vi "FFT -- V2.vi"() -> ()   [LabVIEW 2021]
uses:
  fft -- data win.ctl
  cursor winow sygnal plot.ctl
  cursor window action.ctl
  <vilib>/measure/maspectr.llb/FFT Power Spectrum for N Chan.vi
  <vilib>/measure/NI_MAPro.lvlib
panel:
  in  "landscape":enum32{"Page 1", "Page 2"}(tab)
  in  "scan step":dbl=0.0001 format="%#_3p"
  in  "accumulate":bool
  in  "clear":bool
  in  "update":bool
  out "landscape plot":cluster{dbl[], dbl[]}[](graph)
  in  "offset":dbl(slide)=5968.8832085721915 scale=50.0..50000.0 scale format="%#_3p"
  out "N":dbl=1.0
  in  "scan":bool
  in  "Tab Control":enum32{"Page 1", "Page 2"}(tab)
  in  "Input file path":path=path "/Users/arkadyshekhter/Desktop/gdrive/data/Vikram&Shiva&Zoltan--Aug2025/August_2025/082225/p_c4_006_082225.tdms"
  out "FFT Graph":cluster{"f0":dbl, "df":dbl, "magnitude":dbl[]}[](graph)=[{"f0"=0.0, "df"=323.0255868567349, "magnitude"=array[4691 elements]}]
  out "Signal graph":waveform(dbl)[](graph)=[{"t0"=timestamp(-0.009969989999999984 s since 1904-01-01), "dt"=3.3e-07, "Y"=array[333333 elements], "attributes"=variant("Configuration"=variant(string "[Configuration]\nConfiguration.Post-trigger delay = \"-0.010000000000\"\nConfiguration.Post-trigger duration = \"0.10000000000\"\nConfiguration.Rate = \"3030303.0303\"\nConfiguration.Ranges = \"<size(s)=5> 10.000000000 10.000000000 10.000000000 1.0000000000 1.0000000000\"\nConfiguration.Re-name channels.<size(s)> = \"5\"\nConfiguration.Re-name channels 0 = \"Idot\"\nConfiguration.Re-name channels 1 = \"Bdot\"\nConfiguration.Re-name channels 2 = \"Bproj\"\nConfiguration.Re-name channels 3 = \"freq\"\nConfiguration.Re-name channels 4 = \"drive\"\nConfiguration.Active channels = \"0,1,2,5,6\"\nConfiguration.External\\nclock = \"FALSE\"\nConfiguration.Monitor time\\nconstant = \"1.0000000000\"\nConfiguration.Sync = \"TRUE\"\nConfiguration.Lock-in input channel phases = \"<size(s)=0> \"\nConfiguration.Output channels configuration.<size(s)> = \"0\""), "NI_ChannelName"=variant(string "freq"))}]
  in  "Data window":T1={"Start"=58340, "Length"=9381, "Channel numbers"=[0], "Cannel names"=["freq", ""], "Group name"="p"}
  in  "run":bool
  out "dt (sec)":dbl=3.3e-07
  in  "digitiz. freq (Hz)":dbl=3000000.0 format="%#_3p"
  out "win (sec)":dbl=0.003127 format="%#_3p"
  out "time (sec)":dbl=0.020800065 format="%#_3p"
  in  "signal cursor":T2={"left"=0.01944671559633024, "right "=0.02257377719528174, "center"=0.02101024639580599, "window"=0.0031270615989515034, "cursors"=[0, 1, 2], "relative"=0, "absolute"=0, "fixed vertical offset"=0.0, "vertical offset"=0.0, "skew"=0.0, "default window frac"=0.1, "kind"=enum."symmetric", "skew.left"=0.5, "skew.right"=0.5, "wing order"=enum."back", "Plot ref Syg"=refnum}
  out "scan times":dbl[](array[numeric])
  out "XY Graph":cluster{dbl[], dbl[]}(graph)
  # "OR"
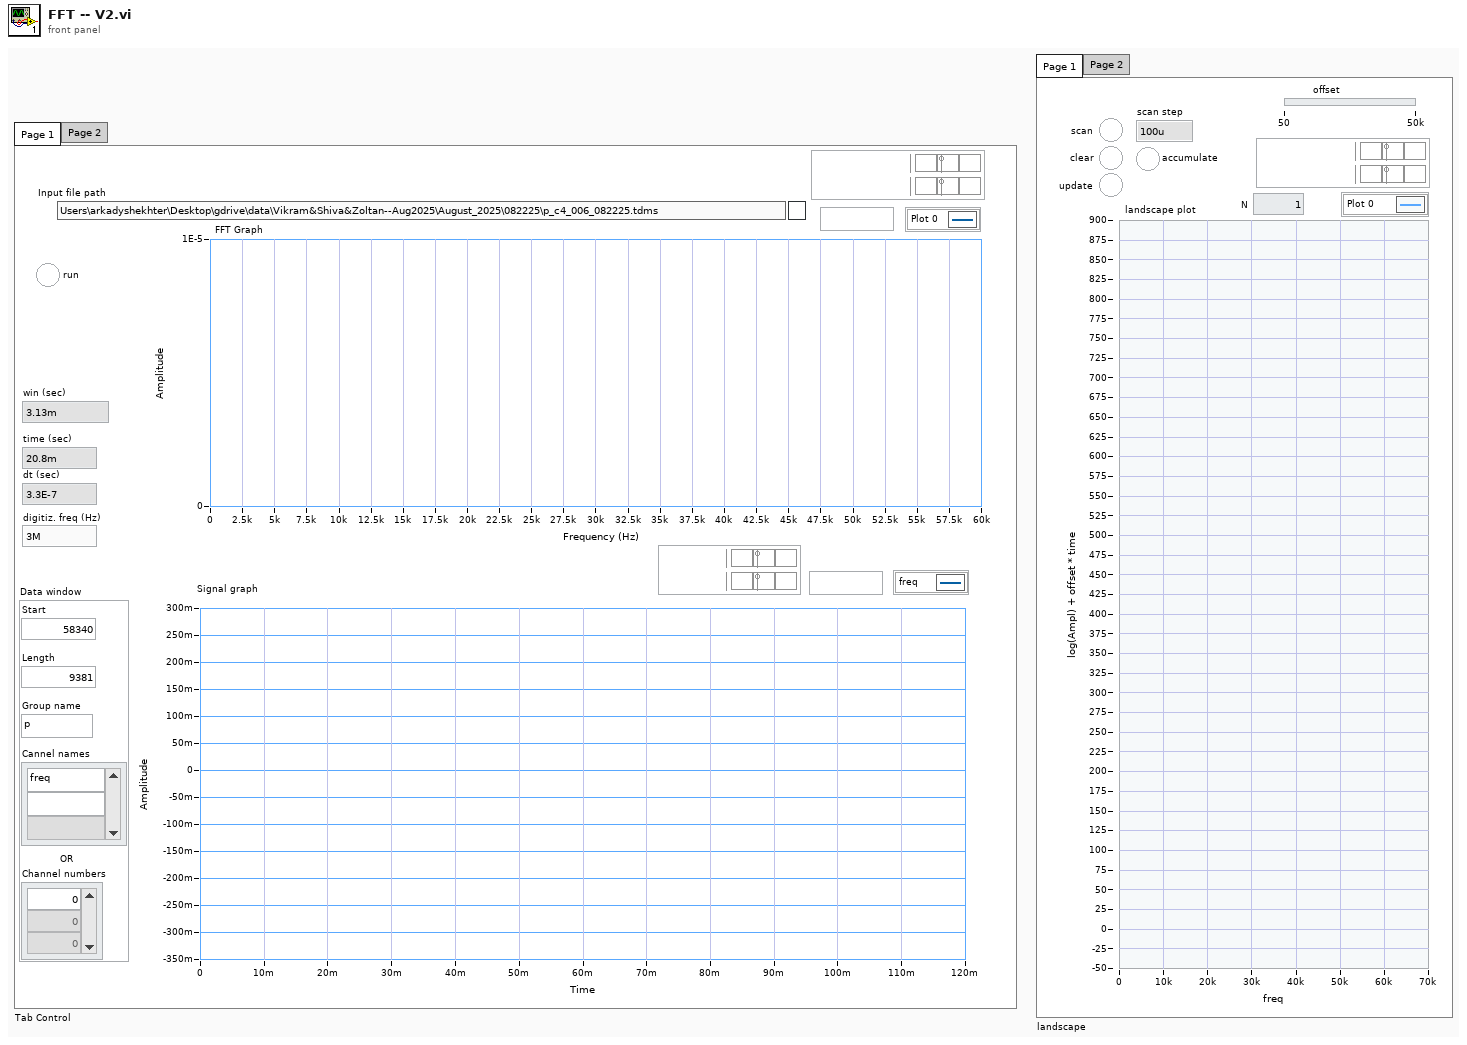
[diagram p1: front panel]
types:
  T1 = typedef "fft -- data win.ctl" = cluster{"Start":i64, "Length":i32, "Channel numbers":i64[], "Cannel names":string[], "Group name":string}
  T2 = typedef "cursor winow sygnal plot.ctl" = cluster{"left":dbl, "right ":dbl, "center":dbl, "window":dbl, "cursors":i32[], "relative":i32, "absolute":i32, "fixed vertical offset":dbl, "vertical offset":dbl, "skew":dbl, "default window frac":dbl, "kind":enum16{"symmetric", "skewed", "fancy"}, "skew.left":dbl, "skew.right":dbl, "wing order":enum16{"forw", "back"}, "Plot ref Syg":refnum<vi>}
  T3 = typedef "cursor window action.ctl" = enum16{"balance", "h. offset change", "cursor moves", "change center", "change window", "init", "check", "reset", "set y to middle", "idle", "-write all Y", "-write left.X", "-write center.X", "-write right.X", "-write all X", "-change center", "-change window", "-change skew", "-read cursor 2", "-read cursor 1", "-read cursor 0", "-read all cursors", "-reset", "-read plot scale", "-set y to middle", "-Q: center.Y is visible", "-Q: window is visible", "-parse center.Y", "-right left from center", "-left move", "-right move", "-set center.Y", "-empty", "-set cursors to default", "-check", "-write center.Y", "-copy cursor 1", "-copy cursor 0", "-copy cursor 2", "move right", "move left", "shrink", "broaden", "skew up", "skew down", "-write plot scale", "zoom X", "change cen&win", "zoom to all data", "color--red", "color--green", "color--yellow", "read", "zoom out", "zoom in", "slide right", "slide left", "set range aspect ratio to 1", "move to window range", "--move to window range"}
  T4 = enum16{"TDMS file", "Tektronics ISF", "BinF file", "ASCII File", "BinH File", "BinW File", "BINARY File"}
  T5 = typedef "eventvkey.ctl" = enum16{"ASCII", "Enter", "Return", "Shift", "Ctrl", "Alt", "Cmd", "Opt", "Caps", "NumLock", "Clear", "Break", "Up", "Down", "Left", "Right", "Insert", "Delete", "Home", "End", "PageUp", "PageDown", "Escape", "Help", "Pause", "ScrollLock", "F1", "F2", "F3", "F4", "F5", "F6", "F7", "F8", "F9", "F10", "F11", "F12", "F13", "F14", "F15", "F16", "F17", "F18", "F19", "F20", "F21", "F22", "F23", "F24", "Play", "VolumeUp", "VolumeDown", "Mute", "Two Byte Char"}
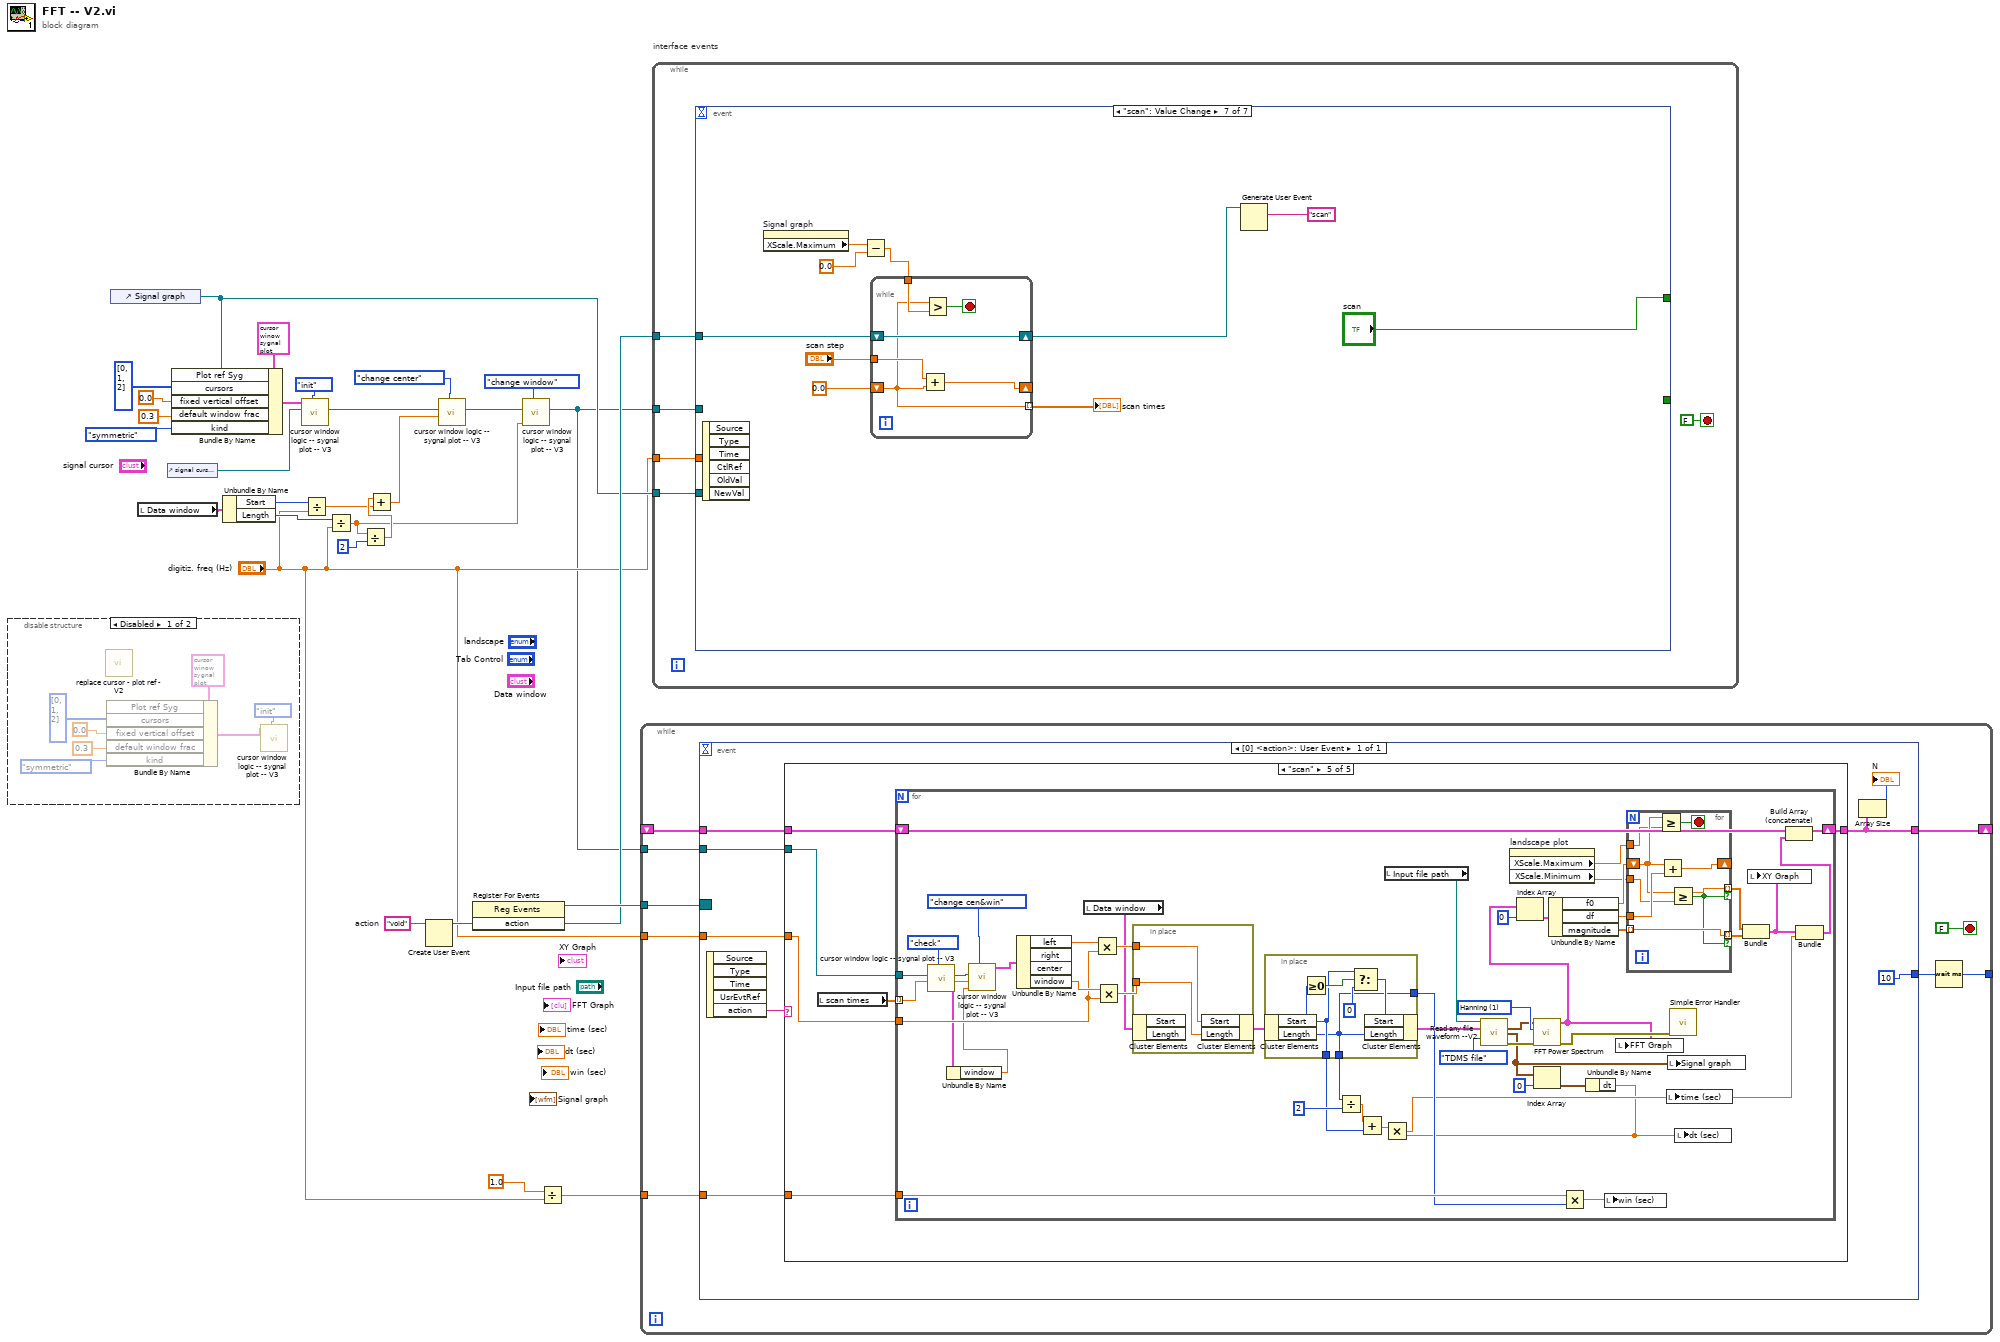
[diagram p0: block diagram]
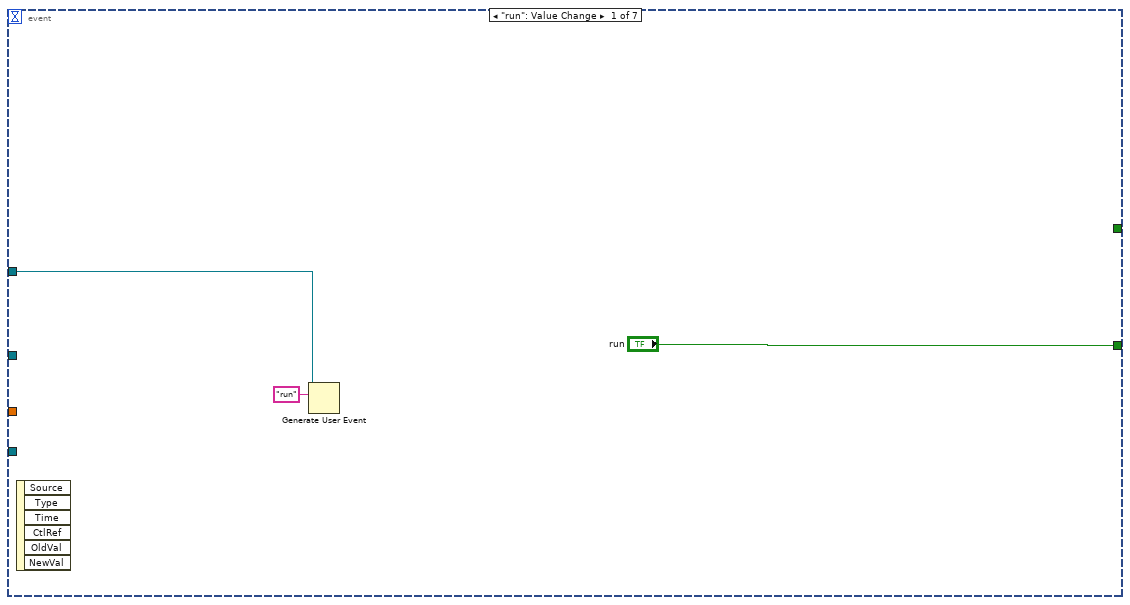
[diagram p3: hidden frame]
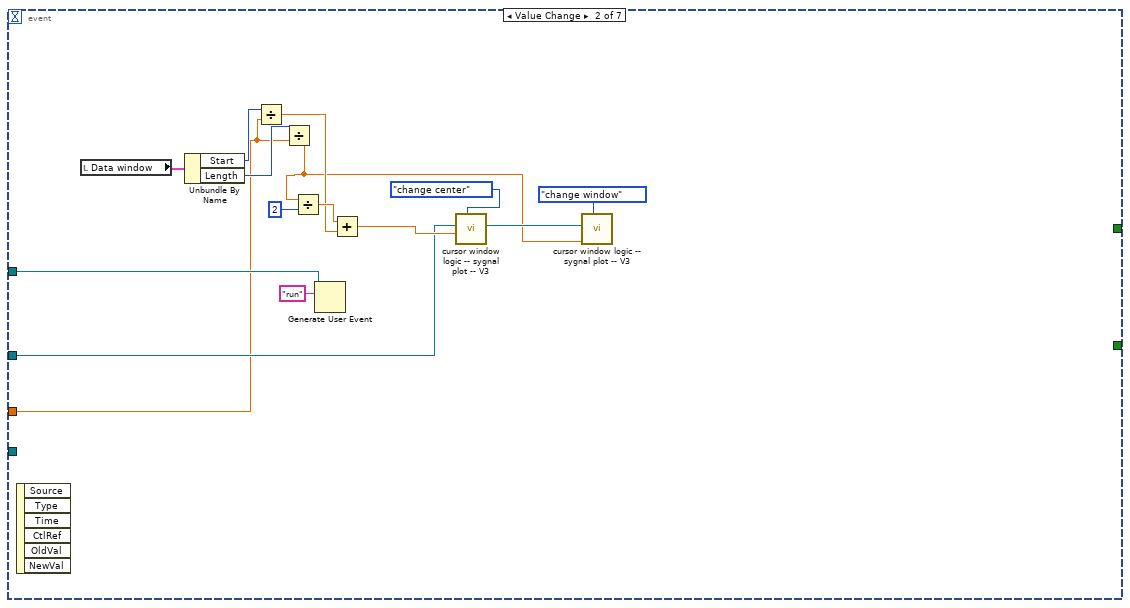
[diagram p4: hidden frame]
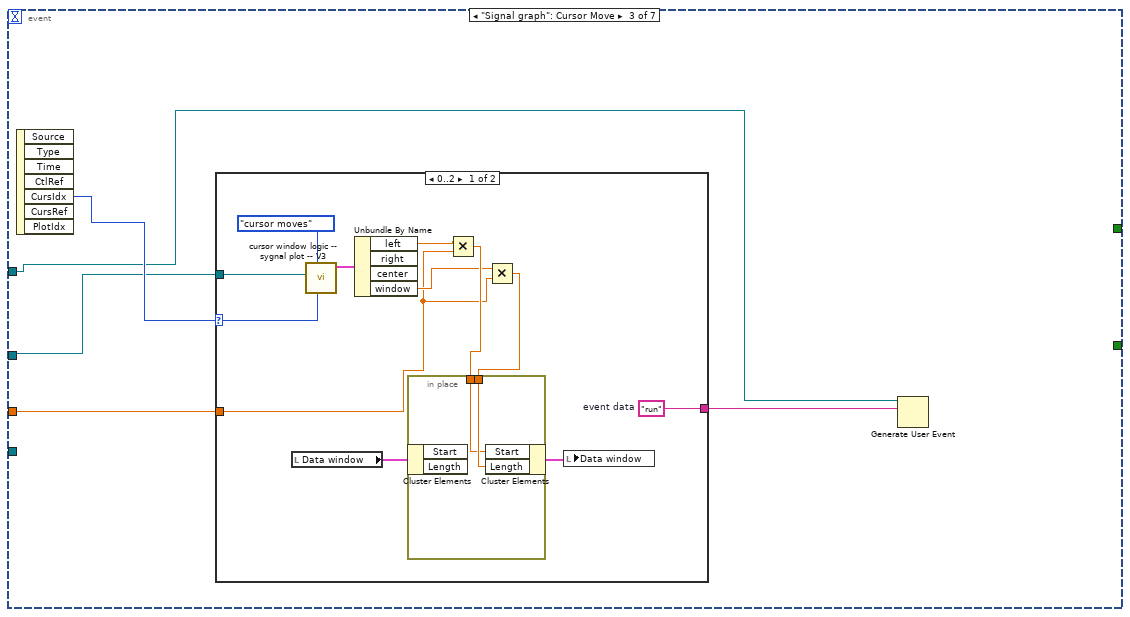
[diagram p5: hidden frame]
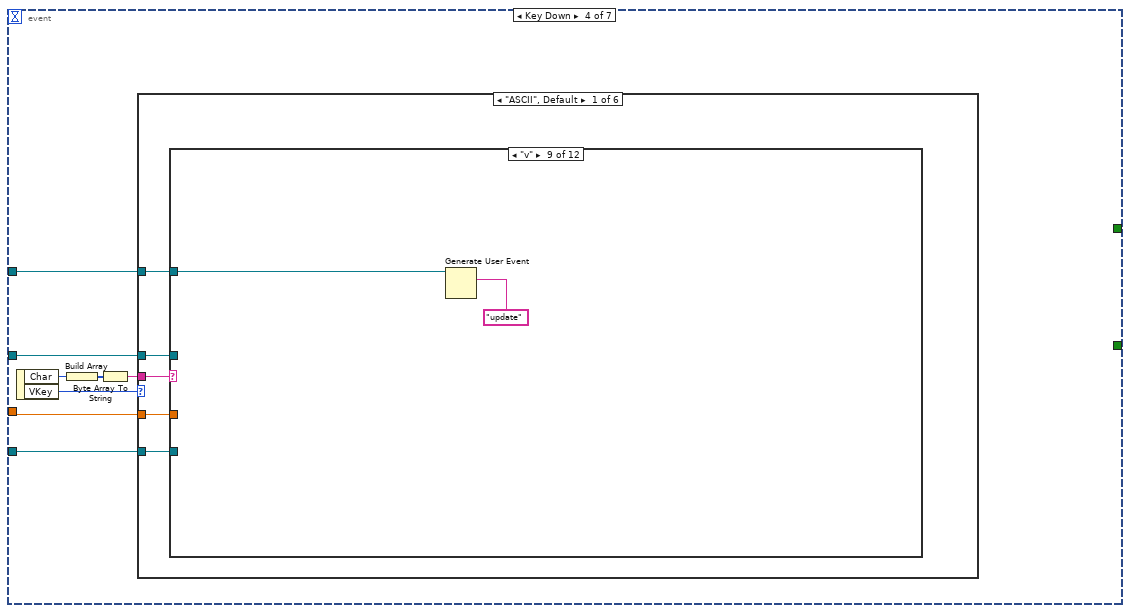
[diagram p7: hidden frame]
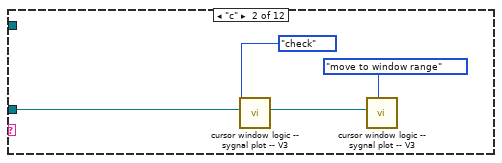
[diagram p9: hidden frame]
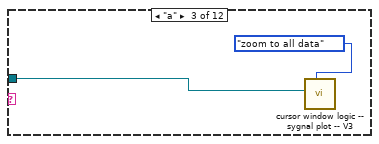
[diagram p10: hidden frame]
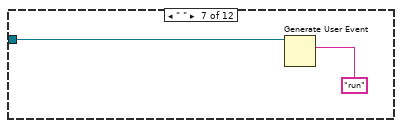
[diagram p14: hidden frame]
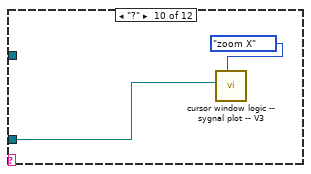
[diagram p16: hidden frame]
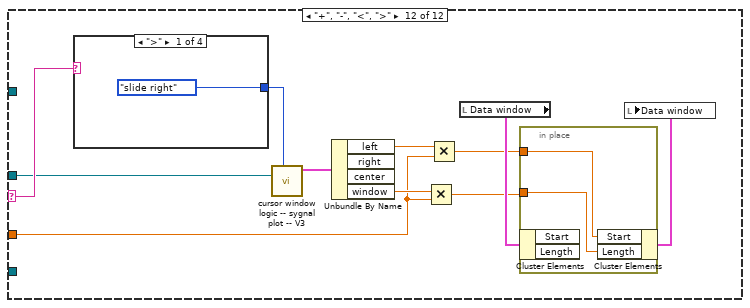
[diagram p18: hidden frame]
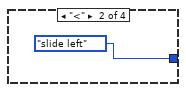
[diagram p19: hidden frame]
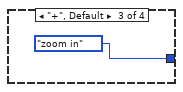
[diagram p20: hidden frame]
diagram:
  w28 = "void"  # action
  n1 = disable-structure shown="Disabled" {
    frame Disabled {
      n2 = call "replace cursor - plot ref - V2.vi"() -> ()  [unwired: 16 in, 4 out]
      n3 = Bundle By Name(cluster=T2 {"left"=2378.60310421286, "right "=2421.6740576496672, "center"=2421.6740576496672, "window"=2421.6740576496672, "cursors"=[], "relative"=0, "absolute"=0, "fixed vertical offset"=2421.6740576496672, "vertical offset"=2421.6740576496672, "skew"=2421.6740576496672, "default window frac"=2421.6740576496672, "kind"=enum."skewed", "skew.left"=2421.6740576496672, "skew.right"=2421.6740576496672, "wing order"=enum."back", "Plot ref Syg"=refnum} ("cursor bracket: All, data window"), "cursors"=i32[] [0, 1, 2], "fixed vertical offset"=0.0, "default window frac"=0.3 ("fixed vertical offset"), "kind"=enum16{"symmetric", "skewed", "fancy"}."symmetric") -> (w29:T2)  [unwired: 1 in]
      n4 = call "cursor window logic -- sygnal plot -- V3.vi"("cursor window action"=cursor_window_action."init", "cursor window init"=w29) -> ()  [unwired: 8 in, 2 out]
    }
    frame Enabled {
    }
  }
  n5 = control-ref of="Signal graph"() -> (w17:refnum<vi>)
  n6 = local read "Data window"() -> (w4:T1)
  n7 = control-ref of="signal cursor ref"() -> (w18:refnum<vi>)
  n8 = Bundle By Name(cluster=T2 {"left"=2378.60310421286, "right "=2421.6740576496672, "center"=2421.6740576496672, "window"=2421.6740576496672, "cursors"=[], "relative"=0, "absolute"=0, "fixed vertical offset"=2421.6740576496672, "vertical offset"=2421.6740576496672, "skew"=2421.6740576496672, "default window frac"=2421.6740576496672, "kind"=enum."skewed", "skew.left"=2421.6740576496672, "skew.right"=2421.6740576496672, "wing order"=enum."back", "Plot ref Syg"=refnum} ("cursor bracket: All, data window"), "Plot ref Syg"=w17, "cursors"=i32[] [0, 1, 2], "fixed vertical offset"=0.0, "default window frac"=0.3 ("fixed vertical offset"), "kind"=enum16{"symmetric", "skewed", "fancy"}."symmetric") -> (w21:T2)
  n9 = Unbundle By Name(w4) -> ("Start"=w5:i64, "Length"=w8:i32)
  n10 = call "cursor window logic -- sygnal plot -- V3.vi"("cursor window action"=cursor_window_action."init", "cursor window IN"=w18, "cursor window init"=w21) -> ("cursor window OUT"=w3:refnum<vi>)  [unwired: 7 in, 1 out]
  n11 = Divide(x=w5, y="digitiz. freq (Hz)") -> (x/y=w7:dbl)
  n12 = Divide(x=w8, y="digitiz. freq (Hz)") -> (x/y=w6:dbl)
  n13 = Divide(x=w6, y=2) -> (x/y=w10:dbl)
  n14 = Add(x=w10, y=w7) -> (x+y=w9:dbl)
  n15 = Create User Event(user event datatype=w28) -> (user event=w26:refnum<user-event>)  [unwired: 1 in, 1 out]
  n16 = call "cursor window logic -- sygnal plot -- V3.vi"("cursor window action"=cursor_window_action."change center", "center"=w9, "cursor window IN"=w3) -> ("cursor window OUT"=w12:refnum<vi>)  [unwired: 7 in, 1 out]
  n17 = register-events(w26) -> (reference out=w27:refnum<event-registration>)  [unwired: 2 in, 1 out]
  n18 = call "cursor window logic -- sygnal plot -- V3.vi"("cursor window action"=cursor_window_action."change window", "window"=w6, "cursor window IN"=w12) -> ("cursor window OUT"=w1:refnum<vi>)  [unwired: 7 in, 1 out]
  n19 = Divide(x=1.0, y="digitiz. freq (Hz)") -> (x/y=w15:dbl)
  n20 = while {
    tunnel: w27 -> [w43]
    tunnel: [w42] -> _
    tunnel: w15 -> [w40]
    shift-right: [w38] -> _
    shift-left: _ -> [w39]
    tunnel: "digitiz. freq (Hz)" -> [w37]
    tunnel: w1 -> [w36]
    stop <- FALSE stop-if-true
    n21 = event shown="[0] <action>: User Event" {
      selector: w43 -> [_]
      dyn-events: _ -> [_]
      timeout: _ -> [_]
      tunnel: [u32 10 ("milliseconds to wait")] -> w41
      tunnel: w40 -> [w51]
      tunnel: [w47] -> w38
      tunnel: w39 -> [w49]
      tunnel: w37 -> [w46]
      tunnel: w36 -> [w45]
      event User Event {
        n22 = event-data() -> ("action"=w50:string)  [unwired: 1 in, 4 out]
        n23 = case shown="\"scan\"" w50 {
          tunnel: w51 -> [_ _ _ w93 w136]
          tunnel: [w53 w57 w62 w84 w131] -> w47
          tunnel: w49 -> [w53 _ w62 w85 w135]
          tunnel: w46 -> [_ _ _ _ w134]
          tunnel: w45 -> [_ _ _ _ w133]
          frame "False", Default {
          }
          frame "clear" {
            w58 = dbl[] []
            n24 = Bundle(w58, w58) -> (w56:cluster{dbl[], dbl[]})  [unwired: 1 in]
            n25 = Bundle(w56, 0.0) -> (w54:cluster{cluster{dbl[], dbl[]}, dbl})  [unwired: 1 in]
            n26 = Build Array(w54) -> (w57:cluster{cluster{dbl[], dbl[]}, dbl}[])
          }
          frame "update" {
            n27 = for {
              tunnel: w62 -> [w76] mode=indexing
              tunnel: "offset" -> [w70]
              tunnel: [w74] -> w59 mode=indexing
              n28 = Unbundle(w76) -> (w73:cluster{dbl[], dbl[]}, w71:dbl)
              n29 = Multiply(x=w71, y=w70) -> (x*y=w69:dbl)
              n30 = Unbundle(w73) -> (w72:dbl[], w68:dbl[])
              n31 = Natural Logarithm(1:w68) -> (0:w67:dbl[])
              n32 = Add(x=w67, y=w69) -> (x+y=w75:dbl[])
              n33 = Bundle(w72, w75) -> (w74:cluster{dbl[], dbl[]})  [unwired: 1 in]
            }
            "landscape plot" <- w59
            n34 = Array Size(array=w59) -> (size(s)=w61:i32)
            n35 = Decrement(x=w61) -> (x-1=w60:i32)
            n36 = for {
              N: w60 -> [_]
              i -> [w65]
              n37 = property on="landscape plot" class="XYGraph (strict)"("Active Plot"=w65) -> (error out=w64:errorcluster)  [unwired: 2 in, 1 out]
              n38 = property on="landscape plot" class="XYGraph (strict)"(error in=w64, "Plot.Plot Color"=u32 5875967) -> ()  [unwired: 1 in, 2 out]
            }
          }
          frame "run" {
            w100 = u32 1 items=["Rectangle"=0, "Hanning"=1, "Hamming"=2, "Blackman-Harris"=3, "Exact Blackman"=4, "Blackman"=5, "Flat Top"=6, "4 Term B-Harris "=7, "7 Term B-Harris"=8, "Low Sidelobe"=9, "Blackman Nuttall"=11, "Triangle"=30, "Bartlett-Hanning"=31, "Bohman"=32, "Parzen"=33, "Welch"=34, "Kaiser"=60, "Dolph-Chebyshev"=61, "Gaussian"=62] ("Window")
            n39 = local read "Data window"() -> (w86:T1)
            n40 = in-place {
              in-place-border: [w126] -> w92
              in-place-border: [w127] -> w88
              in-place-border: [w126] -> w91
              n41 = in-place-cluster #1(w86) -> ("Start"=w127:i64, "Length"=w126:i32)
              n42 = Greater Or Equal To 0?(x=w127) -> (x >= 0?=w130:bool)
              n43 = Select(t=w127, s=w130, f=i64 0 ("Start")) -> (s? t:f=w129:i64)
              n44 = in-place-cluster #1("Start"=w129, "Length"=w126) -> (w94:T1)
            }
            n45 = Divide(x=w91, y=2) -> (x/y=w89:dbl)
            n46 = Add(x=w89, y=w88) -> (x+y=w87:dbl)
            n47 = local read "Input file path"() -> (w82:path)
            n48 = call "Read any file waveform --V2.vi"("Input file path"=w82, "Data window IN"=w94, "Data File Type"=T4."TDMS file") -> ("Data out"=w97:waveform(dbl)[], "All Data out"=w77:waveform(dbl)[], "error out"=w101:errorcluster)  [unwired: 7 in, 3 out]
            n49 = call-poly <vilib>:"FFT Power Spectrum.vi"("error in (no error)"=w101, "window"=w100, "time signals"=w97) -> ("error out"=w98:errorcluster, "power spectra"=w81:cluster{"f0":dbl, "df":dbl, "magnitude":dbl[]}[])  [unwired: 3 in, 4 out]
            n50 = Index Array(array=w77, index=0) -> (element=w95:waveform(dbl))
            n51 = Multiply(x=w93, y=w92) -> (x*y=w78:dbl)
            n52 = Unbundle By Name(w95) -> ("dt"=w79:dbl)
            n53 = Multiply(x=w87, y=w79) -> (x*y=w80:dbl)
            n54 = case shown="True" "accumulate" {
              tunnel: w81 -> [_ w117]
              tunnel: w85 -> [w102 w109]
              tunnel: [w102 w108] -> w84
              tunnel: w80 -> [_ w107]
              frame False {
              }
              frame True {
                n55 = property on="landscape plot" class="XYGraph (strict)"() -> ("XScale.Maximum"=w104:dbl, "XScale.Minimum"=w105:dbl)  [unwired: 2 in, 2 out]
                n56 = Index Array(array=w117, index=0) -> (element=w115:cluster{"f0":dbl, "df":dbl, "magnitude":dbl[]})
                n57 = Unbundle By Name(w115) -> ("f0"=w113:dbl, "df"=w112:dbl, "magnitude"=w114:dbl[])
                n58 = for {
                  tunnel: w114 -> [w123] mode=indexing
                  tunnel: [w123] -> w110 mode=indexing if=w118
                  shift-right: [w125] -> _
                  shift-left: w113 -> [w121]
                  tunnel: [w121] -> w111 mode=indexing if=w118
                  tunnel: w112 -> [w124]
                  tunnel: w105 -> [w122]
                  tunnel: w104 -> [w120]
                  stop <- w119 stop-if-true
                  n59 = Greater Or Equal?(x=w121, y=w120) -> (x >= y?=w119:bool)
                  n60 = Add(x=w121, y=w124) -> (x+y=w125:dbl)
                  n61 = Greater Or Equal?(x=w121, y=w122) -> (x >= y?=w118:bool)
                }
                n62 = Bundle(w111, w110) -> (w103:cluster{dbl[], dbl[]})  [unwired: 1 in]
                n63 = local write "XY Graph"(w103) -> ()
                n64 = Bundle(w103, w107) -> (w106:cluster{cluster{dbl[], dbl[]}, dbl})  [unwired: 1 in]
                n65 = Build Array (concatenate)(w109, w106) -> (w108:cluster{cluster{dbl[], dbl[]}, dbl}[])
              }
            }
            n66 = local write "win (sec)"(w78) -> ()
            n67 = local write "FFT Graph"(w81) -> ()
            n68 = local write "time (sec)"(w80) -> ()
            n69 = local write "Signal graph"(w77) -> ()
            n70 = call <vilib>:"Simple Error Handler.vi"("error in (no error)"=w98) -> ()  [unwired: 4 in, 5 out]
            n71 = local write "dt (sec)"(w79) -> ()
          }
          frame "scan" {
            n72 = local read "scan times"() -> (w132:dbl[])
            n73 = for {
              tunnel: w136 -> [w177]
              tunnel: w134 -> [w146]
              tunnel: w133 -> [w143]
              tunnel: w132 -> [w138] mode=indexing
              shift-right: [w137] -> w131
              shift-left: w135 -> [w170]
              w184 = u32 1 items=["Rectangle"=0, "Hanning"=1, "Hamming"=2, "Blackman-Harris"=3, "Exact Blackman"=4, "Blackman"=5, "Flat Top"=6, "4 Term B-Harris "=7, "7 Term B-Harris"=8, "Low Sidelobe"=9, "Blackman Nuttall"=11, "Triangle"=30, "Bartlett-Hanning"=31, "Bohman"=32, "Parzen"=33, "Welch"=34, "Kaiser"=60, "Dolph-Chebyshev"=61, "Gaussian"=62] ("Window")
              n74 = call "cursor window logic -- sygnal plot -- V3.vi"("cursor window action"=cursor_window_action."check", "cursor window IN"=w143) -> ("cursor window OUT"=w142:refnum<vi>, "cursor window out"=w140:T2)  [unwired: 8 in]
              n75 = Unbundle By Name(w140) -> ("window"=w139:dbl)
              n76 = call "cursor window logic -- sygnal plot -- V3.vi"("cursor window action"=cursor_window_action."change cen&win", "window"=w139, "center"=w138, "cursor window IN"=w142) -> ("cursor window out"=w151:T2)  [unwired: 6 in, 1 out]
              n77 = Unbundle By Name(w151) -> ("left"=w150:dbl, "window"=w148:dbl)  [unwired: 2 out]
              n78 = local read "Data window"() -> (w145:T1)
              n79 = Multiply(x=w150, y=w146) -> (x*y=w149:dbl)
              n80 = Multiply(x=w148, y=w146) -> (x*y=w147:dbl)
              n81 = in-place {
                in-place-border: w147 -> [w187]
                in-place-border: w149 -> [w186]
                n82 = in-place-cluster #2(w145) -> ()  [unwired: 2 out]
                n83 = in-place-cluster #2("Start"=w186, "Length"=w187) -> (w144:T1)
              }
              n84 = in-place {
                in-place-border: [w188] -> w176
                in-place-border: [w189] -> w172
                in-place-border: [w188] -> w175
                n85 = in-place-cluster #3(w144) -> ("Start"=w189:i64, "Length"=w188:i32)
                n86 = Greater Or Equal To 0?(x=w189) -> (x >= 0?=w192:bool)
                n87 = Select(t=w189, s=w192, f=i64 0 ("Start")) -> (s? t:f=w191:i64)
                n88 = in-place-cluster #3("Start"=w191, "Length"=w188) -> (w178:T1)
              }
              n89 = Divide(x=w175, y=2) -> (x/y=w173:dbl)
              n90 = Add(x=w173, y=w172) -> (x+y=w171:dbl)
              n91 = local read "Input file path"() -> (w169:path)
              n92 = call "Read any file waveform --V2.vi"("Input file path"=w169, "Data window IN"=w178, "Data File Type"=T4."TDMS file") -> ("Data out"=w181:waveform(dbl)[], "All Data out"=w164:waveform(dbl)[], "error out"=w185:errorcluster)  [unwired: 7 in, 3 out]
              n93 = property on="landscape plot" class="XYGraph (strict)"() -> ("XScale.Maximum"=w154:dbl, "XScale.Minimum"=w155:dbl)  [unwired: 2 in, 2 out]
              n94 = call-poly <vilib>:"FFT Power Spectrum.vi"("error in (no error)"=w185, "window"=w184, "time signals"=w181) -> ("error out"=w182:errorcluster, "power spectra"=w168:cluster{"f0":dbl, "df":dbl, "magnitude":dbl[]}[])  [unwired: 3 in, 4 out]
              n95 = Index Array(array=w168, index=0) -> (element=w162:cluster{"f0":dbl, "df":dbl, "magnitude":dbl[]})
              n96 = Index Array(array=w164, index=0) -> (element=w179:waveform(dbl))
              n97 = Unbundle By Name(w162) -> ("f0"=w160:dbl, "df"=w159:dbl, "magnitude"=w161:dbl[])
              n98 = Multiply(x=w177, y=w176) -> (x*y=w165:dbl)
              n99 = Unbundle By Name(w179) -> ("dt"=w166:dbl)
              n100 = Multiply(x=w171, y=w166) -> (x*y=w167:dbl)
              n101 = local write "win (sec)"(w165) -> ()
              n102 = local write "FFT Graph"(w168) -> ()
              n103 = for {
                tunnel: w161 -> [w198] mode=indexing
                tunnel: [w198] -> w157 mode=indexing if=w193
                shift-right: [w200] -> _
                shift-left: w160 -> [w196]
                tunnel: [w196] -> w158 mode=indexing if=w193
                tunnel: w159 -> [w199]
                tunnel: w155 -> [w197]
                tunnel: w154 -> [w195]
                stop <- w194 stop-if-true
                n104 = Greater Or Equal?(x=w196, y=w195) -> (x >= y?=w194:bool)
                n105 = Add(x=w196, y=w199) -> (x+y=w200:dbl)
                n106 = Greater Or Equal?(x=w196, y=w197) -> (x >= y?=w193:bool)
              }
              n107 = local write "time (sec)"(w167) -> ()
              n108 = local write "Signal graph"(w164) -> ()
              n109 = call <vilib>:"Simple Error Handler.vi"("error in (no error)"=w182) -> ()  [unwired: 4 in, 5 out]
              n110 = local write "dt (sec)"(w166) -> ()
              n111 = Bundle(w158, w157) -> (w153:cluster{dbl[], dbl[]})  [unwired: 1 in]
              n112 = local write "XY Graph"(w153) -> ()
              n113 = Bundle(w153, w167) -> (w156:cluster{cluster{dbl[], dbl[]}, dbl})  [unwired: 1 in]
              n114 = Build Array (concatenate)(w170, w156) -> (w137:cluster{cluster{dbl[], dbl[]}, dbl}[])
            }
          }
        }
        n115 = Array Size(array=w47) -> (size(s)=→"N":i32)
      }
    }
    n116 = Wait (ms)(milliseconds to wait=w41) -> (millisecond timer value=w42:u32)
  }
  n117 = while "interface events" {
    tunnel: w26 -> [w204]
    tunnel: w17 -> [w203]
    tunnel: w1 -> [w202]
    tunnel: "digitiz. freq (Hz)" -> [w201]
    stop <- FALSE stop-if-true
    n118 = event shown="[6] \"scan\": Value Change" {
      selector: _ -> [_ _ _ _ _ _ _]
      dyn-events: _ -> [_ _ _ _ _ _ _]
      timeout: _ -> [_ _ _ _ _ _ _]
      tunnel: ["run" _ _ _ _ _ _] -> _
      tunnel: w204 -> [w207 w223 w225 w246 w304 w307 w315]
      tunnel: w203 -> [_ _ _ w245 _ _ _]
      tunnel: w202 -> [_ w214 w227 w244 _ _ _]
      tunnel: w201 -> [_ w209 w224 w243 _ _ _]
      tunnel: [_ _ _ _ "update" "clear" "scan"] -> _
      event "run": Value Change {
        n119 = event-data() -> ()  [unwired: 1 in, 6 out]
        n120 = Generate User Event(user event=w207, event data cluster="run" ("event data")) -> ()  [unwired: 2 in, 2 out]
      }
      event Value Change {
        n121 = event-data() -> ()  [unwired: 1 in, 6 out]
        n122 = local read "Data window"() -> (w218:T1)
        n123 = Unbundle By Name(w218) -> ("Start"=w210:i64, "Length"=w213:i32)
        n124 = Divide(x=w210, y=w209) -> (x/y=w212:dbl)
        n125 = Divide(x=w213, y=w209) -> (x/y=w211:dbl)
        n126 = Divide(x=w211, y=2) -> (x/y=w216:dbl)
        n127 = Generate User Event(user event=w223, event data cluster="run" ("event data")) -> ()  [unwired: 2 in, 2 out]
        n128 = Add(x=w216, y=w212) -> (x+y=w215:dbl)
        n129 = call "cursor window logic -- sygnal plot -- V3.vi"("cursor window action"=cursor_window_action."change center", "center"=w215, "cursor window IN"=w214) -> ("cursor window OUT"=w219:refnum<vi>)  [unwired: 7 in, 1 out]
        n130 = call "cursor window logic -- sygnal plot -- V3.vi"("cursor window action"=cursor_window_action."change window", "window"=w211, "cursor window IN"=w219) -> ()  [unwired: 7 in, 2 out]
      }
      event "Signal graph": Cursor Move {
        n131 = event-data() -> ("CursIdx"=w228:i32)  [unwired: 1 in, 6 out]
        n132 = case shown="0..2" w228 {
          selector: w228 -> [w239 _]
          tunnel: w227 -> [w237 _]
          tunnel: [w234 _] -> w226
          tunnel: w224 -> [w230 _]
          frame 0..2 {
            w234 = "run"  # event data
            n133 = local read "Data window"() -> (w236:T1)
            n134 = call "cursor window logic -- sygnal plot -- V3.vi"("CursIdx"=w239, "cursor window action"=cursor_window_action."cursor moves", "cursor window IN"=w237) -> ("cursor window out"=w238:T2)  [unwired: 7 in, 1 out]
            n135 = Unbundle By Name(w238) -> ("left"=w233:dbl, "window"=w231:dbl)  [unwired: 2 out]
            n136 = Multiply(x=w233, y=w230) -> (x*y=w232:dbl)
            n137 = Multiply(x=w231, y=w230) -> (x*y=w229:dbl)
            n138 = in-place {
              in-place-border: w229 -> [w242]
              in-place-border: w232 -> [w241]
              n139 = in-place-cluster #4(w236) -> ()  [unwired: 2 out]
              n140 = in-place-cluster #4("Start"=w241, "Length"=w242) -> (w235:T1)
            }
            n141 = local write "Data window"(w235) -> ()
          }
          frame 3, Default {
          }
        }
        n142 = Generate User Event(user event=w225, event data cluster=w226) -> ()  [unwired: 2 in, 2 out]
      }
      event Key Down {
        n143 = event-data() -> ("Char"=w248:i16, "VKey"=w250:T5)  [unwired: 1 in]
        n144 = Build Array(w248) -> (w249:i16[])
        n145 = Byte Array To String(unsigned byte array=w249) -> (string=w247:string)
        n146 = case shown="\"ASCII\", Default" w250 {
          selector: w250 -> [_ _ _ _ _ w297]
          tunnel: w247 -> [w255 _ _ _ _ _]
          tunnel: w246 -> [w254 _ _ _ _ w285]
          tunnel: w245 -> [w253 _ _ _ _ _]
          tunnel: w244 -> [w252 _ _ _ _ w296]
          tunnel: w243 -> [w251 _ _ _ _ w289]
          frame "ASCII", Default {
            n147 = case shown="\"v\"" w255 {
              selector: w255 -> [_ _ _ _ _ _ _ _ _ _ _ w277]
              tunnel: w254 -> [_ _ _ _ _ _ w262 _ w264 _ _ _]
              tunnel: w253 -> [_ _ _ _ _ _ _ _ _ _ _ _]
              tunnel: w252 -> [_ w258 w260 _ _ _ _ _ _ w266 _ w276]
              tunnel: w251 -> [_ _ _ _ _ _ _ _ _ _ _ w268]
              frame "0", Default {
              }
              frame "c" {
                n148 = call "cursor window logic -- sygnal plot -- V3.vi"("cursor window action"=cursor_window_action."check", "cursor window IN"=w258) -> ("cursor window OUT"=w257:refnum<vi>)  [unwired: 8 in, 1 out]
                n149 = call "cursor window logic -- sygnal plot -- V3.vi"("cursor window action"=cursor_window_action."move to window range", "cursor window IN"=w257) -> ()  [unwired: 8 in, 2 out]
              }
              frame "a" {
                n150 = call "cursor window logic -- sygnal plot -- V3.vi"("cursor window action"=cursor_window_action."zoom to all data", "cursor window IN"=w260) -> ()  [unwired: 8 in, 2 out]
              }
              frame "s" {
              }
              frame "~" {
              }
              frame "l" {
              }
              frame " " {
                n151 = Generate User Event(user event=w262, event data cluster="run" ("event data")) -> ()  [unwired: 2 in, 2 out]
              }
              frame "e" {
              }
              frame "v" {
                n152 = Generate User Event(user event=w264, event data cluster="update" ("event data")) -> ()  [unwired: 2 in, 2 out]
              }
              frame "?" {
                n153 = call "cursor window logic -- sygnal plot -- V3.vi"("cursor window action"=cursor_window_action."zoom X", "cursor window IN"=w266) -> ()  [unwired: 8 in, 2 out]
              }
              frame ",", "." {
              }
              frame "+", "-", "<", ">" {
                n154 = case shown="\">\"" w277 {
                  tunnel: [cursor_window_action."slide right" ("cursor window action") cursor_window_action."slide left" ("cursor window action") cursor_window_action."zoom in" ("cursor window action") cursor_window_action."zoom out" ("cursor window action")] -> w278
                  frame ">" {
                  }
                  frame "<" {
                  }
                  frame "+", Default {
                  }
                  frame "-" {
                  }
                }
                n155 = call "cursor window logic -- sygnal plot -- V3.vi"("cursor window action"=w278, "cursor window IN"=w276) -> ("cursor window out"=w273:T2)  [unwired: 8 in, 1 out]
                n156 = Unbundle By Name(w273) -> ("left"=w272:dbl, "window"=w270:dbl)  [unwired: 2 out]
                n157 = Multiply(x=w270, y=w268) -> (x*y=w269:dbl)
                n158 = Multiply(x=w272, y=w268) -> (x*y=w271:dbl)
                n159 = local read "Data window"() -> (w274:T1)
                n160 = in-place {
                  in-place-border: w269 -> [w280]
                  in-place-border: w271 -> [w279]
                  n161 = in-place-cluster #5(w274) -> ()  [unwired: 2 out]
                  n162 = in-place-cluster #5("Start"=w279, "Length"=w280) -> (w275:T1)
                }
                n163 = local write "Data window"(w275) -> ()
              }
            }
          }
          frame "PageUp" {
          }
          frame "Enter" {
          }
          frame "Caps" {
          }
          frame "PageDown" {
          }
          frame "Up".."Right" {
            n164 = case shown="\"Right\"" w297 {
              tunnel: [cursor_window_action."broaden" ("cursor window action") cursor_window_action."shrink" ("cursor window action") cursor_window_action."move left" ("cursor window action") cursor_window_action."move right" ("cursor window action")] -> w295
              frame "Up", Default {
              }
              frame "Down" {
              }
              frame "Left" {
              }
              frame "Right" {
              }
            }
            n165 = local read "Data window"() -> (w292:T1)
            n166 = call "cursor window logic -- sygnal plot -- V3.vi"("cursor window action"=w295, "cursor window IN"=w296) -> ("cursor window out"=w294:T2)  [unwired: 8 in, 1 out]
            n167 = Unbundle By Name(w294) -> ("left"=w291:dbl, "window"=w290:dbl)  [unwired: 2 out]
            n168 = Multiply(x=w290, y=w289) -> (x*y=w288:dbl)
            n169 = Multiply(x=w291, y=w289) -> (x*y=w287:dbl)
            n170 = in-place {
              in-place-border: w288 -> [w299]
              in-place-border: w287 -> [w298]
              n171 = in-place-cluster #6(w292) -> ()  [unwired: 2 out]
              n172 = in-place-cluster #6("Start"=w298, "Length"=w299) -> (w293:T1)
            }
            n173 = local write "Data window"(w293) -> ()
            n174 = Generate User Event(user event=w285, event data cluster="run" ("event data")) -> ()  [unwired: 2 in, 2 out]
          }
        }
      }
      event "offset", "update": Value Change {
        n175 = event-data() -> ()  [unwired: 1 in, 6 out]
        n176 = Generate User Event(user event=w304, event data cluster="update" ("event data")) -> ()  [unwired: 2 in, 2 out]
      }
      event "clear": Value Change {
        n177 = event-data() -> ()  [unwired: 1 in, 6 out]
        n178 = Generate User Event(user event=w307, event data cluster="clear" ("event data")) -> ()  [unwired: 2 in, 2 out]
      }
      event "scan": Value Change {
        n179 = event-data() -> ()  [unwired: 1 in, 6 out]
        n180 = property on="Signal graph" class="WFGraph (strict)"() -> ("XScale.Maximum"=w313:dbl)  [unwired: 2 in, 2 out]
        n181 = Subtract(x=w313, y=0.0) -> (x-y=w311:dbl)
        n182 = while {
          shift-right: [w325] -> _
          shift-left: 0.0 -> [w320]
          tunnel: "scan step" -> [w323]
          tunnel: [w320] -> w310 mode=indexing
          shift-right: [w324] -> w314
          shift-left: w315 -> [w324]
          tunnel: w311 -> [w322]
          stop <- w321 stop-if-true
          n183 = Add(x=w323, y=w320) -> (x+y=w325:dbl)
          n184 = Greater?(x=w320, y=w322) -> (0:w321:bool)
        }
        "scan times" <- w310
        n185 = Generate User Event(user event=w314, event data cluster="scan" ("event data")) -> ()  [unwired: 2 in, 2 out]
      }
    }
  }
